vi "SetPersonData.vi"(0 "reference in":refnum<class "MyTestClass.lvclass">, 1 "Name":string, 2 "Address":string, 3 "City":string, 5 "error in (no error)":errorcluster) -> (14 "reference out":refnum<class "MyTestClass.lvclass">, 19 "error out":errorcluster)   [LabVIEW 2020, in "MyTestClass.lvclass"]
uses:
  MyTestClass.lvclass
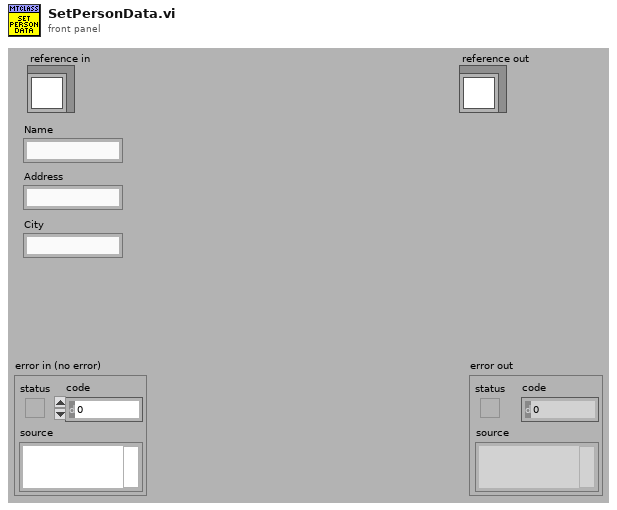
[diagram p1: front panel]
types:
  T1 = typedef "MyTestClass.lvclass/ObjectAttributesRef.ctl" = refnum<data-value>
  T2 = typedef "MyTestClass.lvclass/ObjectAttributes.ctl" = cluster{"Name":string, "Address":string, "City":string}
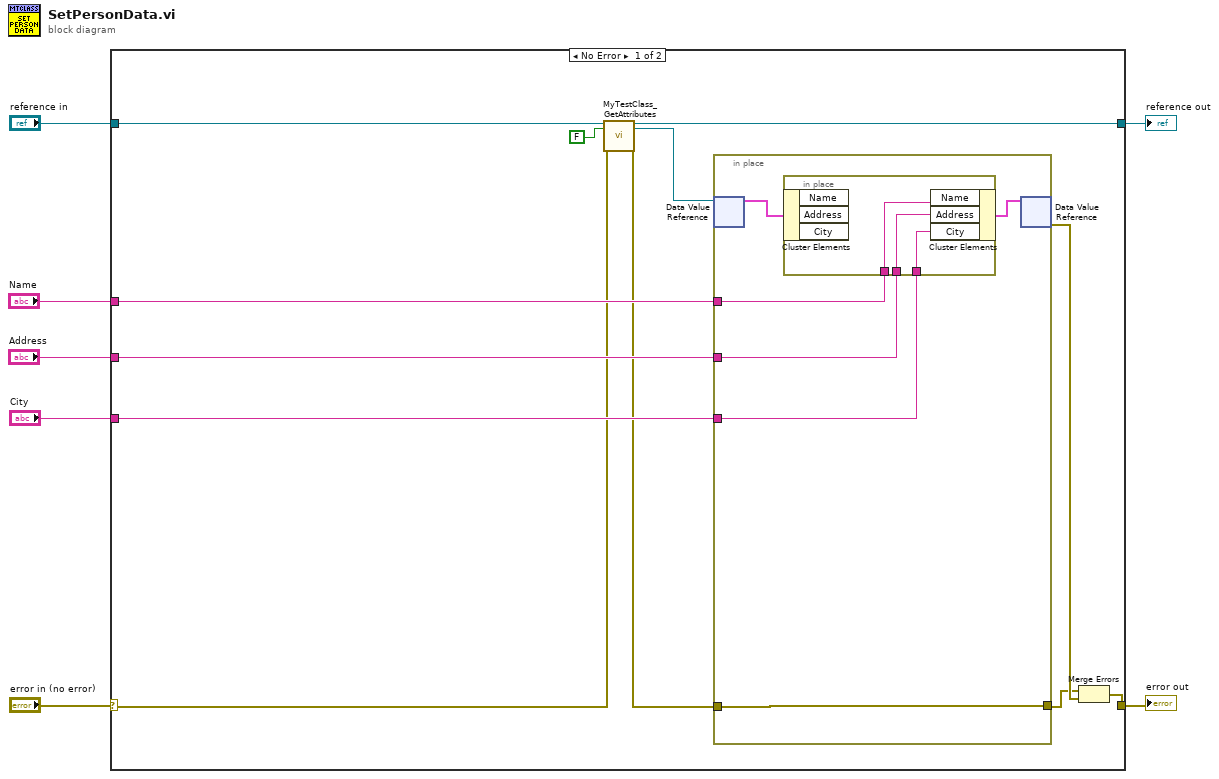
[diagram p0: block diagram]
diagram:
  n1 = case shown="No Error" "error in (no error)" {
    selector: "error in (no error)" -> [w11 w30]
    tunnel: [w19 w30] -> w6
    tunnel: [w12 w29] -> w4
    tunnel: "reference in" -> [w13 w29]
    tunnel: "Name" -> [w16 _]
    tunnel: "Address" -> [w15 _]
    tunnel: "City" -> [w14 _]
    frame No Error {
      n2 = call "MyTestClass_GetAttributes.vi"("reference in"=w13, "return data? (T)"=FALSE, "error in (no error)"=w11) -> ("reference out"=w12:refnum<class "MyTestClass.lvclass">, "attributes ref"=w9:T1, "error out"=w10:errorcluster)  [unwired: 13 in, 1 out]
      n3 = in-place {
        in-place-border: w10 -> [w23]
        in-place-border: [w23] -> w17
        in-place-border: w16 -> [w22]
        in-place-border: w15 -> [w21]
        in-place-border: w14 -> [w20]
        n4 = in-place-dvr #1(w9) -> (w24:T2)  [unwired: 1 out]
        n5 = in-place {
          in-place-border: w22 -> [w28]
          in-place-border: w21 -> [w27]
          in-place-border: w20 -> [w26]
          n6 = in-place-cluster #2(w24) -> ()  [unwired: 3 out]
          n7 = in-place-cluster #2("Name"=w28, "Address"=w27, "City"=w26) -> (w25:T2)
        }
        n8 = in-place-dvr #1(w25) -> (w18:errorcluster)  [unwired: 1 out]
      }
      n9 = Merge Errors(w17, w18) -> (w19:errorcluster)
    }
    frame Error {
    }
  }
  "error out" <- w6
  "reference out" <- w4
